vi "Populate Graves.vi"(8 "Error In":errorcluster, 11 "State In":T1) -> (0 "Error Out":errorcluster, 3 "State Out":T1)   [LabVIEW 2017, in "Graveyard.lvlib"]
uses:
  Graveyard.lvlib
  State.ctl
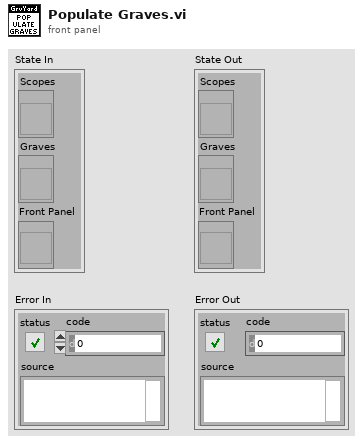
[diagram p1: front panel]
types:
  T1 = typedef "Graveyard.lvlib/State.ctl" = cluster{"Scopes":refnum<vi>, "Graves":refnum<vi>, "Front Panel":refnum<vi>}
  T2 = enum8{"Enabled", "Disabled", "Disabled and Grayed Out"}
  T3 = typedef "Graveyard.lvlib/VI Information.ctl" = cluster{"App Info":T4, "Name":string, "Path":path}
  T4 = typedef "Graveyard.lvlib/Application Information.ctl" = cluster{"Project":string, "Target":string}
  T5 = typedef "Graveyard.lvlib/VI Bookmark.ctl" = cluster{"Bookmark Info":cluster{"Bookmark ID":u32, "Bookmark Tag":string, "Label Text":string}, "VI Info":T3}
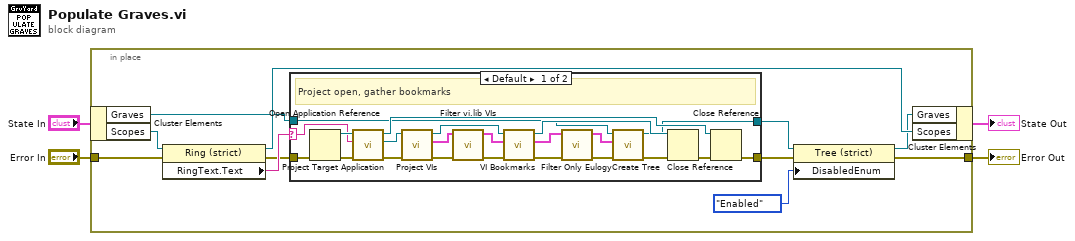
[diagram p0: block diagram]
diagram:
  n1 = in-place {
    in-place-border: "Error In" -> [w13]
    in-place-border: [w8] -> w1
    n2 = in-place-cluster #1("State In") -> ("Graves"=w9:refnum<vi>, "Scopes"=w15:refnum<vi>)
    n3 = property class="Ring (strict)"(reference=w15, error in=w13) -> (reference out=w14:refnum<vi>, error out=w11:errorcluster, "RingText.Text"=w12:string)
    n4 = case shown="Default" w12 {
      selector: w12 -> [w34 _]
      tunnel: w11 -> [w37 w39]
      tunnel: [w33 w39] -> w10
      tunnel: w9 -> [w20 w38]
      tunnel: [w18 w38] -> w7
      frame Default {
        # "Project open, gather bookmarks"
        n5 = Open Application Reference(8:w37) -> (0:w35:errorcluster, 3:w36:refnum<vi>)  [unwired: 3 in]
        n6 = call "Project Target Application.vi"("Error In"=w35, "Project Name"=w34, "App In"=w36) -> ("Error Out"=w31:errorcluster, "Project Target App"=w30:refnum<vi>, "App Out"=w32:refnum<vi>)  [unwired: 6 in]
        n7 = call "Project VIs.vi"("Error In"=w31, "Proejct Target App In"=w30) -> ("Error Out"=w27:errorcluster, "VIs"=w28:T3[], "Project Target App Out"=w24:refnum<vi>)  [unwired: 7 in]
        n8 = call "Filter vi.lib VIs.vi"("Error In"=w27, "VIs In"=w28) -> ("Error Out"=w26:errorcluster, "VIs Out"=w25:T3[])  [unwired: 8 in]
        n9 = call "VI Bookmarks.vi"("Error In"=w26, "VIs"=w25, "Project Target App In"=w24) -> ("Error Out"=w21:errorcluster, "VI Bookmarks"=w22:T5[], "Project Target App Out"=w23:refnum<vi>)  [unwired: 6 in]
        n10 = call "Filter Only Eulogy.vi"("Error In"=w21, "VI Bookmarks"=w22) -> ("Error Out"=w19:errorcluster, "Eulogy Bookmarks"=w16:T5[])  [unwired: 8 in]
        n11 = call "Create Tree.vi"("Error In"=w19, "Graves"=w16, "TreeControl In"=w20) -> ("Error Out"=w17:errorcluster, "TreeControl Out"=w18:refnum<vi>)  [unwired: 7 in]
        n12 = Close Reference(reference=w23, error in (no error)=w17) -> (error out=w29:errorcluster)
        n13 = Close Reference(reference=w32, error in (no error)=w29) -> (error out=w33:errorcluster)
      }
      frame "Main Application Instance" {
        # "No open projects, so no bookmarks to gather"
      }
    }
    n14 = property class="Tree (strict)"(reference=w7, error in=w10, "DisabledEnum"=T2."Enabled" ("Disabled")) -> (reference out=w6:refnum<vi>, error out=w8:errorcluster)
    n15 = in-place-cluster #1("Graves"=w6, "Scopes"=w14) -> (→"State Out":T1)
  }
  "Error Out" <- w1
